vi "Data Log Refresh.vi"(8 "error in (no error)":errorcluster, 11 "Data Cluster":T1) -> (0 "error out":errorcluster)   [LabVIEW 2025]
uses:
  controls/LAB-IQ UI Data.ctl
  Traction Loop/Traction Receipe Enum.ctl
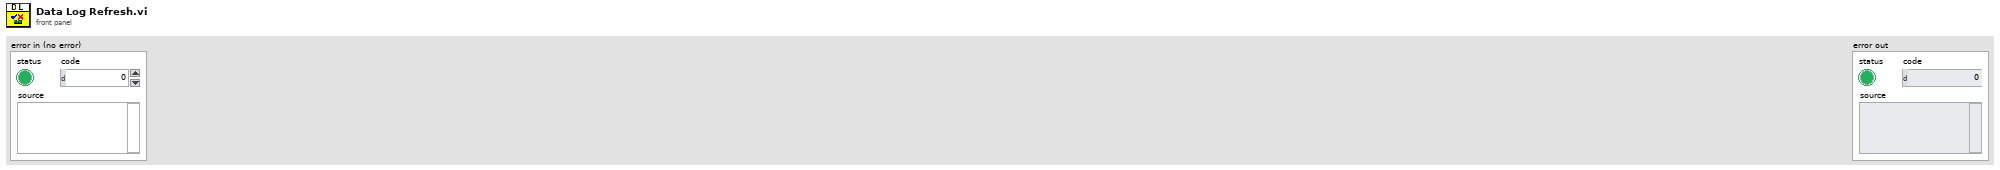
[diagram p1: front panel]
types:
  T1 = typedef "LAB-IQ UI Data.ctl" = cluster{"Main Home Screen":cluster{"GUI":refnum<vi>, "Platform Settings":refnum<vi>, "Configure":refnum<vi>, "Home":refnum<vi>, "EXIT":refnum<vi>, "service 2":refnum<vi>, "MainPage":refnum<vi>, "Analysis":refnum<vi>}, "Platform Settings":cluster{"mm/s  Surge":refnum<vi>, "Drive Error":refnum<vi>, "Disable Axis Jog Soft Limits":refnum<vi>, "mm/s  Sway":refnum<vi>, "Sway and Surge COM Status":refnum<vi>, "Heave COM Status":refnum<vi>, "Enable Platform":refnum<vi>, "Surge Forward Main":refnum<vi>, "Sway Right Main":refnum<vi>, "Sway Left Main":refnum<vi>, "Heave Down Main":refnum<vi>, "Heave Up main":refnum<vi>, "mm/s Heave":refnum<vi>, "mm/sec":refnum<vi>, "mm":refnum<vi>, "Surge Backward Main":refnum<vi>}, "Analysis Screen":cluster{"Analysis Home":refnum<vi>, "Surface Analysis":refnum<vi>, "Imaging":refnum<vi>, "Image Analysis":refnum<vi>, "Post Analysis":refnum<vi>}, "Config Screen":cluster{"Select Load Head":refnum<vi>, "Notes :":refnum<vi>, "FILE":refnum<vi>, "Sample ID :":refnum<vi>, "Operator ID :":refnum<vi>, "Operator Name :":refnum<vi>, "Auto":refnum<vi>}, "Motion Module":cluster{"zNL":refnum<vi>, "NL disp":refnum<vi>, "Rotary Tab":refnum<vi>, "Motion Direction:  3":refnum<vi>, "E.Velocity 2":refnum<vi>, "e.v/ssr 2":refnum<vi>, "Enter Fixed E.Velocity 2":refnum<vi>, "Enter Final SRR 2":refnum<vi>, "Enter initial SRR 2":refnum<vi>, "Enter Fixed SRR 2":refnum<vi>, "Enter the Final E.Velocity (m/s) 2":refnum<vi>, "Enter initial E.Velocity (m/s) 2":refnum<vi>, "Final Speed (RPM) 3":refnum<vi>, "Initial Speed (RPM) 2":refnum<vi>, "Enter the Final Velocity (m/s) 3":refnum<vi>, "Enter initial Velocity (m/s)  3":refnum<vi>, "Ramp Up 2":refnum<vi>, "TEST SELECTION":refnum<vi>, "SPEED SELECTION : ":refnum<vi>, "Angular Oscillation Set":refnum<vi>, "Traction":refnum<vi>, "Step Speed":refnum<vi>, "StepTable For Load-Speed":refnum<vi>, "StepTable For Speed":refnum<vi>, "Surge Forward MM":refnum<vi>, "Surge Backward MM":refnum<vi>, "M3 Image":refnum<vi>, "String 39":refnum<vi>, "Sway Left MM":refnum<vi>, "Sway Right MM":refnum<vi>, "Disable Axis Jog Soft Limits":refnum<vi>, "mm":refnum<vi>, "Heave Down MM":refnum<vi>, "Heave Up MM":refnum<vi>, "Wear Track Diameter (mm)":refnum<vi>, "Set WTD":refnum<vi>, "HomeScratch":refnum<vi>, "HomeRot":refnum<vi>, "PlaceModule":refnum<vi>, "Enter the Angle (Deg)":refnum<vi>, "Enter the Frequency (Hz)":refnum<vi>, "Motion Mode:":refnum<vi>, "LR Sway":refnum<vi>, "Rot Hor":refnum<vi>, "Scratch":refnum<vi>, "LR Cam":refnum<vi>, "MMBack":refnum<vi>, "MMNext":refnum<vi>, "Rot Ver":refnum<vi>, "Rotary Module Selection":refnum<vi>, "calculate rotary":refnum<vi>, "SPEED SELECTION : rotary":refnum<vi>, "Import 2":refnum<vi>, "Save 2":refnum<vi>, "File Path :  2":refnum<vi>, "String 45":refnum<vi>, "StepTable For Speed 3":refnum<vi>, "Enter the Speed(mm/sec)":refnum<vi>, "Enter the Speed(RPM)":refnum<vi>, "Enter Scratch Speed (mm/s):":refnum<vi>, "SwaySpeed Set":refnum<vi>, "Scartch Offset":refnum<vi>, "Motion type:":refnum<vi>, "HomeScratch 2":refnum<vi>, "Enter Scratch length (mm):":refnum<vi>, "Wear Track Diameter":refnum<vi>, "Rotary Speed Exced":refnum<vi>, "Scratch Mode":refnum<vi>, "No of Scratch":refnum<vi>}, "Environmental control":cluster{"Humidity  Status  3":refnum<vi>, "Low Temp  Status  2":refnum<vi>, "TK4 status 2":refnum<vi>, "Stage Temperature":refnum<vi>, "Sample Temperature":refnum<vi>, "Humidity (Amb)":refnum<vi>, "Clear List":refnum<vi>, "Add to list":refnum<vi>, "Wear":refnum<vi>, "Vibration":refnum<vi>, "Humidity (Chamber)":refnum<vi>, "Temperature (Chamber)":refnum<vi>, "ECR ":refnum<vi>, "Temperature (Amb)":refnum<vi>, "Microphone":refnum<vi>, "Acoustic Emission 3":refnum<vi>, "SNext":refnum<vi>, "APBack":refnum<vi>, "Enter the Temperature (°C):":refnum<vi>, "Enter the Stage \nTemperature (°C):":refnum<vi>, "Enter the Humidity (%Rh):":refnum<vi>, "Low Temp":refnum<vi>, "High Temp":refnum<vi>, "Humidity":refnum<vi>, "Sensors Picked":refnum<vi>}, "About Screen":cluster{"Password":refnum<vi>, "Home Service":refnum<vi>, "Advanced Setting":refnum<vi>, "About Tab":refnum<vi>, "ECR Port:":refnum<vi>, "Ramp Port:":refnum<vi>, "Installation/Replacement completed":refnum<vi>, "Loahead":refnum<vi>, "Heave and Surge COM Port:":refnum<vi>, "Sway COM Port:":refnum<vi>, "Temp Modbus:":refnum<vi>, "Humidity Port:":refnum<vi>, "Edit Gain Constants":refnum<vi>, "Save Gain Constants":refnum<vi>}, "Main Screen":cluster{"Main Screen Tab":refnum<vi>, "Angle and Frequency":refnum<vi>, "Stroke (mm)":refnum<vi>, "Angle (Deg)":refnum<vi>, "Main Speed Tab":refnum<vi>, "MTM MOTOR DISPLAY":refnum<vi>, "Disc Speed (m/sec)":refnum<vi>, "Ball Speed (m/sec)":refnum<vi>, "Disc Speed (RPM)":refnum<vi>, "Ball Speed (RPM)":refnum<vi>, "SPEED TAB":refnum<vi>, "Speed (m/sec)":refnum<vi>, "Set Speed (m/sec)":refnum<vi>, "Speed (RPM)":refnum<vi>, "Set Speed":refnum<vi>, "Time Tab":refnum<vi>, "Time ( HH:MM:SS ) 2":refnum<vi>, "Test Duration":refnum<vi>, "Test Duration 4":refnum<vi>, "TEST CYCLE":refnum<vi>, "TOTAL CYCLES":refnum<vi>, "Set Load (N)":refnum<vi>, "Temp Tabs":refnum<vi>, "Heater":refnum<vi>, "TK4 status":refnum<vi>, "ChamberTemp":refnum<vi>, "SetTmp":refnum<vi>, "Controller  Status":refnum<vi>, "ChamberTemp 2":refnum<vi>, "SetTmp 2":refnum<vi>, "Controller  Status 2":refnum<vi>, "ChamberTemp 3":refnum<vi>, "SetTmp 3":refnum<vi>, "Cooling":refnum<vi>, "Load Communication":refnum<vi>, "Ambient \nTemperature":refnum<vi>, "HumCOMStatus":refnum<vi>, "Ambient\n Humidity":refnum<vi>, "Freq (Hz)":refnum<vi>, "Load En":refnum<vi>, "NLt":refnum<vi>, "zNL 2":refnum<vi>, "Humidity On":refnum<vi>, "humidity disp":refnum<vi>, "Set Humidity":refnum<vi>, "NL disp 2":refnum<vi>, "Humidity On 2":refnum<vi>, "humidity disp 2":refnum<vi>, "Set Humidity 2":refnum<vi>, "NL disp 3":refnum<vi>, "AppLoadSeq scratch":refnum<vi>, "Stop Scratch":refnum<vi>, "ClrLog":refnum<vi>, "Trip Log":refnum<vi>, "STOP":refnum<vi>, "Start Test":refnum<vi>, "Test status":refnum<vi>, "AR Led":refnum<vi>, "Data":refnum<vi>, "Health":refnum<vi>, "Sway COM Status":refnum<vi>, "Heave COM Status":refnum<vi>, "Grp Tab":refnum<vi>, "Sub Graph":refnum<vi>, "SD (mm)":refnum<vi>, "Siliding distance Reset Graph":refnum<vi>, "SDGp":refnum<vi>, "Humidity Reset Graph":refnum<vi>, "HumrGp":refnum<vi>, "Acoustic Emission (mV)":refnum<vi>, "Aqucostic Reset Graph":refnum<vi>, "gACQUOS":refnum<vi>, "ECR RESET":refnum<vi>, "ECR":refnum<vi>, "Temperature Reset":refnum<vi>, "Acoustic Emission (mV) 2":refnum<vi>, "Aqucostic Reset Graph 2":refnum<vi>, "gACQUOS 2":refnum<vi>, "ECR RESET 2":refnum<vi>, "ECR 2":refnum<vi>, "Temperature Reset 2":refnum<vi>, "Temperature (deg c)":refnum<vi>, "Speed Reset Graph":refnum<vi>, "Speed Tab":refnum<vi>, "MTM DISC  SPEED":refnum<vi>, "MTM BALL SPEED":refnum<vi>, "speed mm/sec":refnum<vi>, "Hymidity":refnum<vi>, "Humidity Disable trip":refnum<vi>, "CoF Trip  2":refnum<vi>, "Depth Trip":refnum<vi>, "Weart Deapth":refnum<vi>, "Depth Reset Graph":refnum<vi>, "Weart":refnum<vi>, "Depthz":refnum<vi>, "Depth (µm)":refnum<vi>, "WearGp":refnum<vi>, "NL Trip 2":refnum<vi>, "Load pid":refnum<vi>, "Load Disable Trip":refnum<vi>, "Load Reset Graph":refnum<vi>, "NL Display 4":refnum<vi>, "Main Chart 3":refnum<vi>, "BACK":refnum<vi>, "Depth Trip 2":refnum<vi>, "COF TRIP ":refnum<vi>, "Friction Force (N)":refnum<vi>, "FF Reset Graph":refnum<vi>, "FF Disable Trip":refnum<vi>, "FF TRIP":refnum<vi>, "COF Disable Trip":refnum<vi>, "COF Reset Graph":refnum<vi>, "Start Test Temp":refnum<vi>, "zFF":refnum<vi>, "Friction Force (N) Graph":refnum<vi>, "Coefficient of Friction":refnum<vi>, "Scratch Start Test":refnum<vi>, "FF Tab":refnum<vi>, "Cyclic Friction Force (N)":refnum<vi>, "CZ FF":refnum<vi>, "Cyclic Friction Force (N) Graph":refnum<vi>, "Cyclic Coefficient of Friction":refnum<vi>, "Cyclic FF TRIP":refnum<vi>, "Cyclic FF Disable Trip":refnum<vi>, "cyclic COF Disable Trip":refnum<vi>, "cyclic COF TRIP":refnum<vi>, "cyclic COF Reset Graph":refnum<vi>, "Cyclic FF Reset Graph":refnum<vi>, "Test Trip":refnum<vi>, "Multi Scratch Pass":refnum<vi>, "Scratch Start Recording":refnum<vi>}, "Loading":cluster{"Indentation":refnum<vi>, "Reference Sample":refnum<vi>, "Load Cell Communication Slide":refnum<vi>, "com 3":refnum<vi>, "com":refnum<vi>, "DecaForce COM Status":refnum<vi>, "Update":refnum<vi>, "Clear 3":refnum<vi>, "seq":refnum<vi>, "Stribeck table":refnum<vi>, "Stribeck Table  For loading":refnum<vi>, "Loading Mode":refnum<vi>, "Enter the Final Load (N)":refnum<vi>, "Enter the CoF Trip":refnum<vi>, "Enter the Friction Force Trip":refnum<vi>, "Enter the Normal load Trip":refnum<vi>, "Enter the Load  (N)":refnum<vi>, "KiloForce":refnum<vi>, "DecaForce ":refnum<vi>, "MicroForce":refnum<vi>, "LHBack":refnum<vi>, "LHNext":refnum<vi>, "Enter the Loading Rate (N/min)":refnum<vi>, "Message":refnum<vi>, "Warning 2":refnum<vi>, "SSP 0.75":refnum<vi>, "SSP 0.5":refnum<vi>, "SSP 0.3":refnum<vi>, "Warning":refnum<vi>, "gui GIF":refnum<vi>, "Communication is established":refnum<vi>, "AppLoad 4":refnum<vi>, "Multipoint":refnum<vi>, "Load Selection":refnum<vi>}, "PID":cluster{"Ramp":refnum<vi>, "Vertical load (N)":refnum<vi>, "apply load":refnum<vi>, "apply load 2":refnum<vi>, "Enter ByPass Load":refnum<vi>, "Bypass Load":refnum<vi>, "gFF Rot":refnum<vi>}, "Config Parameters":cluster{"Tab Control 3":refnum<vi>, "Tab Control 19":refnum<vi>, "SAMPLES":refnum<vi>, "Re-initilaize":refnum<vi>, "Filter ON/OFF":refnum<vi>, "TracHomeSurgeOffsetCounts 10MM":refnum<vi>, "TracHomeSwayOffsetCounts 10MM":refnum<vi>, "Acoustic Emission:":refnum<vi>, "Apply Filter (FF)":refnum<vi>, "Filter% 2":refnum<vi>, "Apply Filter (Load)":refnum<vi>, "Filter% ":refnum<vi>, "Sway distance (mm)":refnum<vi>, "Surge distance (mm)":refnum<vi>, "DataSavingLoopDelay(ms)":refnum<vi>, "SAVE 2":refnum<vi>, "Enter Distance":refnum<vi>, "Sway Counts:":refnum<vi>, "Distance (mm): 3":refnum<vi>, "Surge Counts:":refnum<vi>, "Distance (mm): 2":refnum<vi>, "Distance (mm):":refnum<vi>, "Heave Counts:":refnum<vi>, "LRMHomeSurgeOffsetCounts":refnum<vi>, "LRMHomeSwayOffsetCounts":refnum<vi>, "TracHomeSurgeOffsetCounts 20MM":refnum<vi>, "TracHomeSwayOffsetCounts 20MM":refnum<vi>, "RotHomeSwayOffsetCounts":refnum<vi>, "RotHomeSurgeOffsetCounts":refnum<vi>, "Heave distance":refnum<vi>, "Zmm":refnum<vi>, "Heave Pulses/mm":refnum<vi>, "Surge Pulses/mm":refnum<vi>, "Sway Pulses/mm":refnum<vi>, "Heave Pitch":refnum<vi>, "Surge Pitch":refnum<vi>, "Sway Pitch":refnum<vi>, "Heave PPR":refnum<vi>, "Surge PPR":refnum<vi>, "Sway PPR":refnum<vi>, "Tab Control 5":refnum<vi>, "Tab Control 14":refnum<vi>, "Tab Control 26":refnum<vi>, "AE":refnum<vi>, "Heave Loop Delay":refnum<vi>, "Heave PID Speed":refnum<vi>, "Surge Jog Speed":refnum<vi>, "Heave Jog Speed":refnum<vi>, "Sway Loop Delay":refnum<vi>, "Sway PID Speed":refnum<vi>, "Sway Jog Speed":refnum<vi>, "DEPTH TRIP VALUE":refnum<vi>, "LOAD TRIP VALUE":refnum<vi>, "DEPTH TRIP   ENABLE":refnum<vi>, "LOAD TRIP  ENABLE":refnum<vi>, "CYCLIC FF TRIP VALUE":refnum<vi>, "FF TRIP VALUE":refnum<vi>, "CYCLIC CoF TRIP VALUE":refnum<vi>, "COF TRIP VALUE":refnum<vi>, "CYCLIC COF TRIP  ENABLE":refnum<vi>, "CYCLIC FF TRIP  ENABLE":refnum<vi>, "FF TRIP  ENABLE":refnum<vi>, "COF TRIP  ENABLE":refnum<vi>, "JOG TRIP LOAD VALUE (N)":refnum<vi>, "Rotary Vertical":refnum<vi>, "Traction":refnum<vi>, "Scratch":refnum<vi>, "LRM CAM":refnum<vi>, "Sway LRM":refnum<vi>, "Rotary Horizontal":refnum<vi>}, "Loading Com Port":cluster{"ClearAll":refnum<vi>, "Mz(Nm)":refnum<vi>, "My(Nm)":refnum<vi>, "Mx(Nm)":refnum<vi>, "Save Dwell":refnum<vi>, "Acq Delay (ms)":refnum<vi>, "Burst Delay (ms)":refnum<vi>, "model":refnum<vi>, "SN":refnum<vi>, "FFx(N)":refnum<vi>, "Sensor IP":refnum<vi>, "Port":refnum<vi>, "FFy(N)":refnum<vi>, "Load(N)":refnum<vi>, "delete Handle":refnum<vi>, "Create Handle":refnum<vi>, "ft_data":refnum<vi>, "ft_range":refnum<vi>, "ft_data 2":refnum<vi>, "stop 6":refnum<vi>, "running_flag":refnum<vi>, "ft_udp_handle":refnum<vi>, "get-data-return":refnum<vi>, "get-range-return":refnum<vi>, "zero-return":refnum<vi>, "filter-return":refnum<vi>, "initial-return":refnum<vi>, "deleteHandle-result":refnum<vi>, "Load Cell Temp":refnum<vi>, "Load Cell":refnum<vi>, "ZeroAll":refnum<vi>, "FORCE (N)":refnum<vi>, "TORQUE (N-m)":refnum<vi>, "Load Cell Link":refnum<vi>}, "Heave AND Surge":cluster{"SURGE POSE":refnum<vi>, "error out Read":refnum<vi>, "HEAVE POSE":refnum<vi>, "State":refnum<vi>, "Homed":refnum<vi>, "Sequence ID":refnum<vi>, "error out Write":refnum<vi>, "faultCode":refnum<vi>, "Ack ID":refnum<vi>, "SPEED":refnum<vi>, "Distance":refnum<vi>, "Mode Command":refnum<vi>, "Heave and Surge Read":refnum<vi>, "Read Heave Temp":refnum<vi>, "Spare 15":refnum<vi>, "Spare 14":refnum<vi>, "Spare 13":refnum<vi>, "Spare 12":refnum<vi>, "Spare 11":refnum<vi>, "Spare 10":refnum<vi>, "Spare 9":refnum<vi>, "Spare 8":refnum<vi>, "Spare 7":refnum<vi>, "Spare 4":refnum<vi>, "Spare 3":refnum<vi>, "Spare 2":refnum<vi>, "Humidity":refnum<vi>, "Temp":refnum<vi>, "Node Id":refnum<vi>, "Spare 1":refnum<vi>, "SPARE 4":refnum<vi>, "SPARE 3":refnum<vi>, "SPARE 2":refnum<vi>, "SPARE 1":refnum<vi>, "fwMajor":refnum<vi>, "fwMinor":refnum<vi>, "Manual Write":refnum<vi>, "Heave and Surge Write":refnum<vi>, "SPARE 5":refnum<vi>, "Reserved ":refnum<vi>, "SPARE 8":refnum<vi>, "SPARE 6":refnum<vi>, "SPARE 7":refnum<vi>, "SPARE 17":refnum<vi>, "SPARE 16":refnum<vi>, "SPARE 15":refnum<vi>, "SPARE 14":refnum<vi>, "SPARE 13":refnum<vi>, "SPARE 12":refnum<vi>, "SPARE 11":refnum<vi>, "SPARE 10":refnum<vi>, "SPARE 9":refnum<vi>, "System UPTIME":refnum<vi>, "Missed Packets":refnum<vi>, "faultCode Surge Right":refnum<vi>, "faultCode Surge Left":refnum<vi>, "faultCode Heave":refnum<vi>, "UPLINK HEAVE":refnum<vi>, "DOWNLINK HEAVE":refnum<vi>}, "New PID LOGIC":cluster{"Fine Tune Zone":refnum<vi>, "PID SDelay":refnum<vi>, "Max_pos_limit":refnum<vi>, "Min_pos_limit":refnum<vi>, "i_limit":refnum<vi>, "pct_scale":refnum<vi>, "Deadband":refnum<vi>, "Kd":refnum<vi>, "Ki":refnum<vi>, "Kp":refnum<vi>, "Current Position":refnum<vi>, "Set Load":refnum<vi>, "Current Load":refnum<vi>, "Pulse delta":refnum<vi>, "Init Step":refnum<vi>, "Max Step Linit":refnum<vi>, "min_deadband_floor":refnum<vi>, "dynamic_spindle_noise_scalar":refnum<vi>, "min_finetune_floor":refnum<vi>, "filter_alpha":refnum<vi>, "PID":refnum<vi>}, "SWAY ":cluster{"fwMajor":refnum<vi>, "Homed":refnum<vi>, "Rotary POSE":refnum<vi>, "State":refnum<vi>, "SWAY POSE":refnum<vi>, "Ack ID":refnum<vi>, "faultCode":refnum<vi>, "Node Id":refnum<vi>, "fwMinor":refnum<vi>, "Spare 6":refnum<vi>, "Spare 5":refnum<vi>, "Spare 4":refnum<vi>, "Spare 3":refnum<vi>, "Spare 2":refnum<vi>, "Spare 1":refnum<vi>, "Spare 7":refnum<vi>, "SPARE  5":refnum<vi>, "error out Write  SWAY ":refnum<vi>, "error out Read SWAY ":refnum<vi>, "Manual Write SWAY ":refnum<vi>, "SWAY WRITE":refnum<vi>, "SPARE  4":refnum<vi>, "SPARE  3":refnum<vi>, "SPARE 2":refnum<vi>, "SPARE 1":refnum<vi>, "Spare 15":refnum<vi>, "Spare 14":refnum<vi>, "Spare 13":refnum<vi>, "Spare 12":refnum<vi>, "Spare 11":refnum<vi>, "Spare 9":refnum<vi>, "Spare 8":refnum<vi>, "SPEED":refnum<vi>, "Distance":refnum<vi>, "Mode Command":refnum<vi>, "Sequence ID":refnum<vi>, "SWAY READ":refnum<vi>, "Spare 10":refnum<vi>, "Read SWAY Temp":refnum<vi>, "faultCode Sway ":refnum<vi>, "Missed Packets":refnum<vi>, "System UPTIME sway":refnum<vi>, "SPARE 6":refnum<vi>, "SPARE 7":refnum<vi>, "SPARE 9":refnum<vi>, "SPARE 11":refnum<vi>, "SPARE 10":refnum<vi>, "SPARE 8":refnum<vi>, "SPARE 13":refnum<vi>, "SPARE 12":refnum<vi>, "SPARE 17":refnum<vi>, "SPARE 16":refnum<vi>, "SPARE 15":refnum<vi>, "SPARE 14":refnum<vi>, "Reserved":refnum<vi>, "faultCode Rotary":refnum<vi>, "UPLINK SWAY":refnum<vi>, "DOWNLINK SWAY":refnum<vi>}, "Analysis Screen":cluster{"Analysis Home":refnum<vi>, "Refresh 2":refnum<vi>, "MEAN 4":refnum<vi>, "SD 4":refnum<vi>, "VARIANCE 4":refnum<vi>, "MEAN  3":refnum<vi>, "SD  3":refnum<vi>, "VARIANCE  3":refnum<vi>, "MEAN 2":refnum<vi>, "SD  2":refnum<vi>, "VARIANCE 2":refnum<vi>, "MEAN":refnum<vi>, "SD":refnum<vi>, "VARIANCE":refnum<vi>, "File 4 Discription":refnum<vi>, "OPEN 4":refnum<vi>, "File Name 4":refnum<vi>, "OPEN 3":refnum<vi>, "File 3 Discription":refnum<vi>, "File Name 3":refnum<vi>, "Y-AXIS":refnum<vi>, "X-AXIS":refnum<vi>, "XY Graph":refnum<vi>, "File Name 2":refnum<vi>, "File Name 1":refnum<vi>, "OPEN 2":refnum<vi>, "OPEN 1":refnum<vi>, "File 1 Discription ":refnum<vi>, "File 2 Discription":refnum<vi>, "Export":refnum<vi>, "File Format":refnum<vi>}, "Traction":cluster{"faultCode Traction 2":refnum<vi>, "faultCode Traction 1":refnum<vi>, "Missed Packets":refnum<vi>, "System UPTIME Traction":refnum<vi>, "SPARE 17":refnum<vi>, "SPARE 16":refnum<vi>, "SPARE 15":refnum<vi>, "SPARE 14":refnum<vi>, "SPARE 13":refnum<vi>, "SPARE 12":refnum<vi>, "SPARE 11":refnum<vi>, "SPARE 10":refnum<vi>, "SPARE 9":refnum<vi>, "SPARE 8":refnum<vi>, "SPARE 7":refnum<vi>, "SPARE 6":refnum<vi>, "Reserved":refnum<vi>, "SPARE  5":refnum<vi>, "Manual Write TRACTION":refnum<vi>, "TRACTION WRITE":refnum<vi>, "SPARE  4":refnum<vi>, "SPARE  3":refnum<vi>, "SPARE 2":refnum<vi>, "SPARE 1":refnum<vi>, "Spare 7":refnum<vi>, "Spare 6":refnum<vi>, "Spare 5":refnum<vi>, "Spare 4":refnum<vi>, "Spare 2":refnum<vi>, "Spare 1":refnum<vi>, "Node Id":refnum<vi>, "Read TRACTION Temp":refnum<vi>, "fwMinor":refnum<vi>, "fwMajor":refnum<vi>, "faultCode":refnum<vi>, "TRACTION POSE":refnum<vi>, "TRACTION POSE 2":refnum<vi>, "Homed":refnum<vi>, "State":refnum<vi>, "Ack ID":refnum<vi>, "SPEED":refnum<vi>, "Distance":refnum<vi>, "Mode Command":refnum<vi>, "Sequence ID":refnum<vi>, "error out Read TRACTION":refnum<vi>, "error out Write  TRACTION":refnum<vi>, "TRACTION READ":refnum<vi>, "Spare 3":refnum<vi>, "Downlink traction":refnum<vi>, "Uplink Traction":refnum<vi>}, "Traction reciepe":cluster{"SRR Sweep Range (%) Stribeck":refnum<vi>, "Traction Receipe":refnum<vi>, "Total Execution Time":refnum<vi>, "Total Steps":refnum<vi>, "Duration / Step (s)  Stribeck":refnum<vi>, "STRIBECK Fixed SRR List (%)":refnum<vi>, "Duration / Step (s) Traction":refnum<vi>, "SRR Sweep Range (%) traction":refnum<vi>, "Rolling Speed (mm/s)":refnum<vi>, "Temperature Stages (°C)":refnum<vi>, "Ball Load (N)":refnum<vi>, "Lubricant Name":refnum<vi>, "Profile File Name":refnum<vi>, "SET entrainment Velocity":refnum<vi>, "Test Array Size":refnum<vi>, "SRR INDEX [ STRIBECK]":refnum<vi>, "Stribeck Size":refnum<vi>, "SET SRR":refnum<vi>, "ELAPSED TIMER ":refnum<vi>, "BALL SET RPM":refnum<vi>, "DISC SET RPM":refnum<vi>, "SET LOAD":refnum<vi>, "TEMPERATURE READ":refnum<vi>, "SET TEMPERATURE":refnum<vi>, "Traction Size":refnum<vi>, "DISC SPEED (rpm)":refnum<vi>, "BALL SPEED (rpm)":refnum<vi>, "BALL WEAR TRACK":refnum<vi>, "DISC WEARTRACK":refnum<vi>, "SRR INDEX [ TRACTION]":refnum<vi>, "Start Index Type":refnum<vi>, "Enum - Menu":refnum<vi>, "Ball (mm/sec)":refnum<vi>, "Disc (mm/sec)":refnum<vi>}, "Traction Control":cluster{"HomeTraction":refnum<vi>, "Demo Mode Display":refnum<vi>, "Traction Message":refnum<vi>, "Traction Step Update Details":refnum<vi>, "Main Tab sequence for selection":refnum<vi>, "Ramp Tab":refnum<vi>, "e.v/ssr":refnum<vi>, "Enter Fixed E.Velocity":refnum<vi>, "Enter Final SRR":refnum<vi>, "Enter initial SRR":refnum<vi>, "Enter Fixed SRR":refnum<vi>, "Enter the Final E.Velocity (m/s)":refnum<vi>, "Enter initial E.Velocity (m/s)":refnum<vi>, "Ball WTD":refnum<vi>, "E.Velocity":refnum<vi>, "Enter the Final Velocity (m/s)":refnum<vi>, "Enter initial Velocity (m/s)":refnum<vi>, "Ramp Up   Disc":refnum<vi>, "Initial DiscSpeed (RPM)":refnum<vi>, "Final Speed (RPM) Ball":refnum<vi>, "Final Speed (RPM)":refnum<vi>, "Initial Speed (RPM) Ball":refnum<vi>, "Enter the Final Velocity (m/s) Ball":refnum<vi>, "Enter initial Velocity (m/s) Ball":refnum<vi>, "Ramp Up":refnum<vi>, "ExceedBallSpeed step":refnum<vi>, "ExceedDiscSpeed":refnum<vi>, "BallSpeed Exceed Indication":refnum<vi>, "Apply":refnum<vi>, "SPEED SELECTION : MTM":refnum<vi>, "SPEED SELECTION : MTM 2":refnum<vi>, "TEST SELECTION (MTM)":refnum<vi>, "MTM Test Selection":refnum<vi>, "File Path Tab":refnum<vi>, "File Path String":refnum<vi>, "Save":refnum<vi>, "Save  2":refnum<vi>, "Import ":refnum<vi>, "File Path :":refnum<vi>, "Step Sequence Indication Tab":refnum<vi>, "Step Sequence Indication":refnum<vi>, "Calculate Step":refnum<vi>, "StepTable":refnum<vi>, "ExceedDiscSpeed  Cinstant Speed":refnum<vi>, "ExceedBallSpeed Constant":refnum<vi>, "TEST SELECTION (MTM) 2":refnum<vi>, "SPEED SELECTION : MTM 3":refnum<vi>, "MTM Test Selection 2":refnum<vi>, "Enter the Speed (m/sec): ":refnum<vi>, "Enter the Speed (m/sec):  2":refnum<vi>, "Enter the Speed (RPM):":refnum<vi>, "Lower Spped ":refnum<vi>, "Upper":refnum<vi>, "Enter the Speed (RPM):Ball":refnum<vi>, "Disc Motion Direction: ":refnum<vi>, "Ball Motion Direction :":refnum<vi>, "Motion Mode: ":refnum<vi>, "Wear Track Diameter (mm) ":refnum<vi>, "Disc Speed Indicator":refnum<vi>, "ExceedBallSpeed":refnum<vi>}, "Acquostic":cluster{"Last Config Rejected ":refnum<vi>, "rx command count":refnum<vi>, "Current Filter Id":refnum<vi>, "Isolated Gain":refnum<vi>, "DAQ Status":refnum<vi>, "error out":refnum<vi>, "error in (no error)":refnum<vi>, "Uplink Packet":refnum<vi>, "data out":refnum<vi>, "Downlink Packet":refnum<vi>, "Gains":refnum<vi>, "Manual Write Acquostic":refnum<vi>, "Acoustic Graphs":refnum<vi>}}
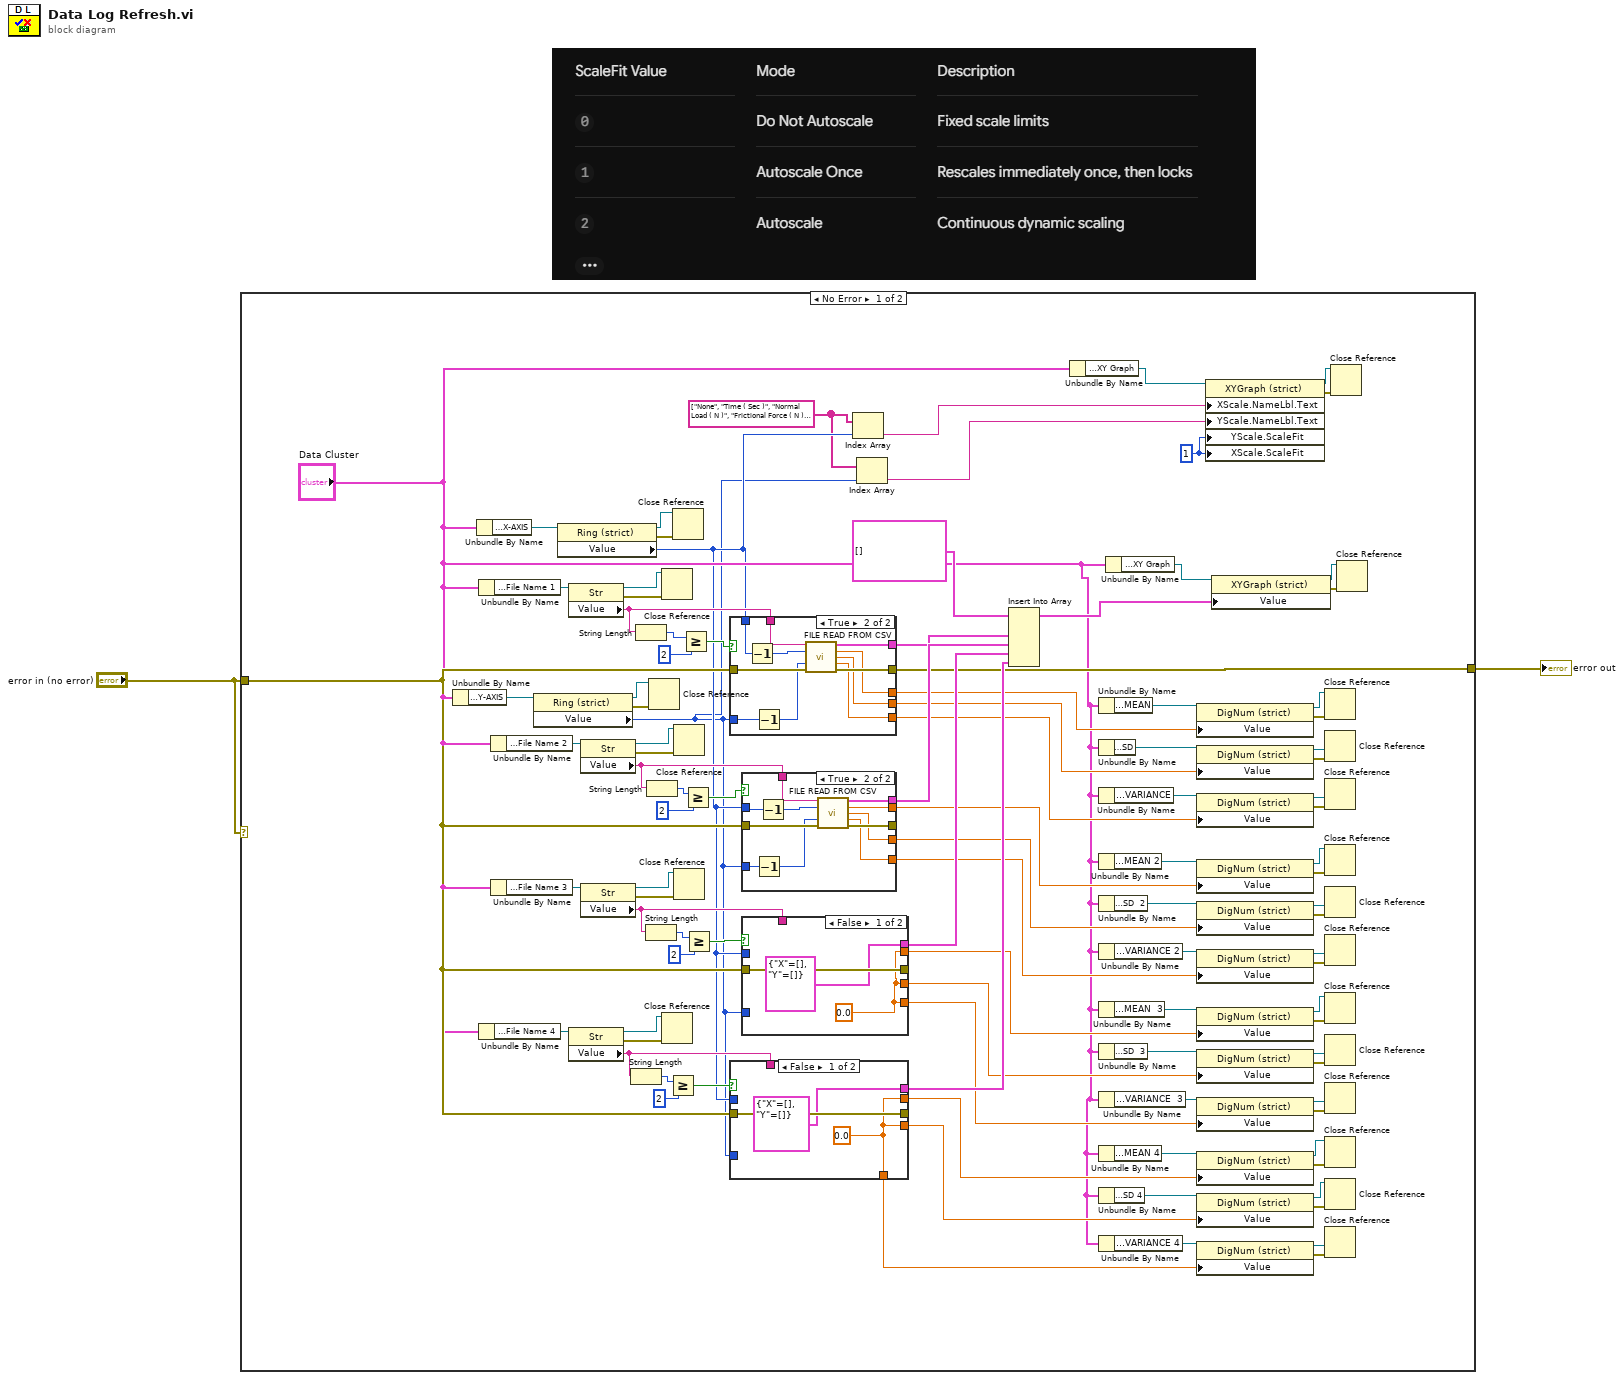
[diagram p0: block diagram]
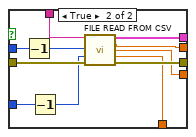
[diagram p2: hidden frame]
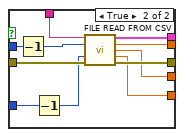
[diagram p3: hidden frame]
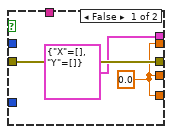
[diagram p4: hidden frame]
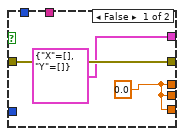
[diagram p5: hidden frame]
diagram:
  n1 = case shown="No Error" "error in (no error)" {
    tunnel: "error in (no error)" -> [w90 _]
    tunnel: [w64 _] -> w2
    frame No Error {
      w3 = u8 1 ("X Scale.Scale Fit")
      w6 = string[] ["None", "Time ( Sec )", "Normal Load ( N )", "Frictional Force ( N )", "Coefficient of Friction", "Depth ( Microns )", "Speed ( RPM )", "Frequency ( Hz )", "Angle ( Degree )", "Cyclic Friction Force ( N )", "Cyclic Co efficient Friction ", "Stage temperature ( Degree celcius )", "Sample temperature ( Degree celcius )", "Stroke Length ( mm )", "Scratch Speed ( mm/sec )", "Amb Humidity ( % Rh ) ", "Amb Temperature (Deg C)", "Acoustic (mV)", "Mx (Nm)", "My (Nm)", "Mz (Nm)", "Humidity ( % Rh )", "Sliding Distance (mm)", "Wear Track Diameter (mm)", "Fx(N)", "Fy(N)", "MTM BallSpeed (RPM)", "MTM DiscSpeed (RPM)", "Entrainment Speed", "Slide Role", "Slip(%)", "Rotary Speed (m/sec)", "MTM Ball Speed (m/sec)", "MTM Disc Speed (m/sec)", "ECR (ohms)"] ("Strings []")
      n2 = Unbundle By Name("Data Cluster") -> ("Analysis Screen.Y-AXIS"=w103:refnum<vi>)
      n3 = Unbundle By Name("Data Cluster") -> ("Analysis Screen.X-AXIS"=w100:refnum<vi>)
      n4 = Unbundle By Name("Data Cluster") -> ("Analysis Screen.File Name 1"=w62:refnum<vi>)
      n5 = Unbundle By Name("Data Cluster") -> ("Analysis Screen.File Name 4"=w84:refnum<vi>)
      n6 = Unbundle By Name("Data Cluster") -> ("Analysis Screen.File Name 2"=w74:refnum<vi>)
      n7 = Unbundle By Name("Data Cluster") -> ("Analysis Screen.File Name 3"=w77:refnum<vi>)
      n8 = property class="Ring (strict)"(reference=w103) -> (reference out=w105:refnum<vi>, error out=w104:errorcluster, "Value"=w5:u16)  [unwired: 1 in]
      n9 = property class="Ring (strict)"(reference=w100) -> (reference out=w102:refnum<vi>, error out=w101:errorcluster, "Value"=w8:u16)  [unwired: 1 in]
      n10 = property class="Str"(reference=w62) -> (reference out=w61:refnum<vi>, error out=w63:errorcluster, "Value"=w65:string)  [unwired: 1 in]
      n11 = property class="Str"(reference=w84) -> (reference out=w83:refnum<vi>, error out=w85:errorcluster, "Value"=w86:string)  [unwired: 1 in]
      n12 = property class="Str"(reference=w74) -> (reference out=w75:refnum<vi>, error out=w73:errorcluster, "Value"=w72:string)  [unwired: 1 in]
      n13 = property class="Str"(reference=w77) -> (reference out=w76:refnum<vi>, error out=w78:errorcluster, "Value"=w79:string)  [unwired: 1 in]
      n14 = String Length(string=w86) -> (length=w87:i32)
      n15 = String Length(string=w65) -> (length=w66:i32)
      n16 = String Length(string=w79) -> (length=w80:i32)
      n17 = String Length(string=w72) -> (length=w71:i32)
      n18 = Close Reference(reference=w105, error in (no error)=w104) -> ()  [unwired: 1 out]
      n19 = Close Reference(reference=w61, error in (no error)=w63) -> ()  [unwired: 1 out]
      n20 = Close Reference(reference=w83, error in (no error)=w85) -> ()  [unwired: 1 out]
      n21 = Greater Or Equal?(x=w87, y=2) -> (x >= y?=w89:bool)
      n22 = Close Reference(reference=w102, error in (no error)=w101) -> ()  [unwired: 1 out]
      n23 = Close Reference(reference=w75, error in (no error)=w73) -> ()  [unwired: 1 out]
      n24 = Close Reference(reference=w76, error in (no error)=w78) -> ()  [unwired: 1 out]
      n25 = Greater Or Equal?(x=w66, y=2) -> (x >= y?=w68:bool)
      n26 = Greater Or Equal?(x=w71, y=2) -> (x >= y?=w69:bool)
      n27 = Greater Or Equal?(x=w80, y=2) -> (x >= y?=w82:bool)
      n28 = case shown="True" w68 {
        tunnel: w90 -> [w150 w161]
        tunnel: [w150 w160] -> w64
        tunnel: w65 -> [_ w159]
        tunnel: [cluster{"X":dbl[], "Y":dbl[]} {"X"=[], "Y"=[]} ("output cluster") w158] -> w95
        tunnel: w8 -> [_ w157]
        tunnel: w5 -> [_ w156]
        tunnel: [w148 w153] -> w51
        tunnel: [w148 w152] -> w50
        tunnel: [w148 w151] -> w49
        frame False {
          w148 = 0.0
        }
        frame True {
          n29 = Decrement(x=w157) -> (x-1=w155:u16)
          n30 = Decrement(x=w156) -> (x-1=w154:u16)
          n31 = call "FILE READ FROM CSV.vi"("File Path"=w159, "X-AXIS"=w155, "Y-AXIS"=w154, "error in (no error)"=w161) -> ("output cluster"=w158:cluster{"X":dbl[], "Y":dbl[]}, "mean"=w153:dbl, "standard deviation"=w152:dbl, "variance"=w151:dbl, "error out"=w160:errorcluster)  [unwired: 7 in]
        }
      }
      n32 = case shown="False" w89 {
        tunnel: w90 -> [w108 w119]
        tunnel: [w108 w118] -> _
        tunnel: w86 -> [_ w117]
        tunnel: [cluster{"X":dbl[], "Y":dbl[]} {"X"=[], "Y"=[]} ("output cluster") w116] -> w98
        tunnel: w8 -> [_ w115]
        tunnel: w5 -> [_ w113]
        tunnel: [w106 w111] -> w15
        tunnel: [w106 w110] -> w14
        tunnel: [w106 w109] -> w13
        frame False {
          w106 = 0.0
        }
        frame True {
          n33 = Decrement(x=w115) -> (x-1=w114:u16)
          n34 = Decrement(x=w113) -> (x-1=w112:u16)
          n35 = call "FILE READ FROM CSV.vi"("File Path"=w117, "X-AXIS"=w114, "Y-AXIS"=w112, "error in (no error)"=w119) -> ("output cluster"=w116:cluster{"X":dbl[], "Y":dbl[]}, "mean"=w111:dbl, "standard deviation"=w110:dbl, "variance"=w109:dbl, "error out"=w118:errorcluster)  [unwired: 7 in]
        }
      }
      n36 = case shown="True" w69 {
        tunnel: w90 -> [w136 w147]
        tunnel: [w136 w146] -> _
        tunnel: w72 -> [_ w145]
        tunnel: [cluster{"X":dbl[], "Y":dbl[]} {"X"=[], "Y"=[]} ("output cluster") w144] -> w96
        tunnel: w8 -> [_ w143]
        tunnel: w5 -> [_ w141]
        tunnel: [w134 w139] -> w39
        tunnel: [w134 w138] -> w38
        tunnel: [w134 w137] -> w37
        frame False {
          w134 = 0.0
        }
        frame True {
          n37 = Decrement(x=w141) -> (x-1=w140:u16)
          n38 = Decrement(x=w143) -> (x-1=w142:u16)
          n39 = call "FILE READ FROM CSV.vi"("File Path"=w145, "X-AXIS"=w142, "Y-AXIS"=w140, "error in (no error)"=w147) -> ("output cluster"=w144:cluster{"X":dbl[], "Y":dbl[]}, "mean"=w139:dbl, "standard deviation"=w138:dbl, "variance"=w137:dbl, "error out"=w146:errorcluster)  [unwired: 7 in]
        }
      }
      n40 = case shown="False" w82 {
        tunnel: w90 -> [w122 w133]
        tunnel: [w122 w132] -> _
        tunnel: w79 -> [_ w131]
        tunnel: [cluster{"X":dbl[], "Y":dbl[]} {"X"=[], "Y"=[]} ("output cluster") w130] -> w97
        tunnel: w8 -> [_ w129]
        tunnel: w5 -> [_ w127]
        tunnel: [w120 w125] -> w27
        tunnel: [w120 w124] -> w26
        tunnel: [w120 w123] -> w25
        frame False {
          w120 = 0.0
        }
        frame True {
          n41 = Decrement(x=w129) -> (x-1=w128:u16)
          n42 = Decrement(x=w127) -> (x-1=w126:u16)
          n43 = call "FILE READ FROM CSV.vi"("File Path"=w131, "X-AXIS"=w128, "Y-AXIS"=w126, "error in (no error)"=w133) -> ("output cluster"=w130:cluster{"X":dbl[], "Y":dbl[]}, "mean"=w125:dbl, "standard deviation"=w124:dbl, "variance"=w123:dbl, "error out"=w132:errorcluster)  [unwired: 7 in]
        }
      }
      n44 = Index Array(array=w6, index=w8) -> (element=w7:string)
      n45 = Index Array(array=w6, index=w5) -> (element=w4:string)
      n46 = Insert Into Array(array=cluster{"Array 2":dbl[], "Array 2":dbl[]}[] [] ("Value"), new element #1=w95, new element #2=w96, new element #3=w97, new element #4=w98) -> (w99:cluster{"Array 2":dbl[], "Array 2":dbl[]}[])  [unwired: 1 in]
      n47 = Unbundle By Name("Data Cluster") -> ("Analysis Screen.XY Graph"=w11:refnum<vi>)
      n48 = Unbundle By Name("Data Cluster") -> ("Analysis Screen.MEAN"=w59:refnum<vi>)
      n49 = Unbundle By Name("Data Cluster") -> ("Analysis Screen.SD"=w56:refnum<vi>)
      n50 = Unbundle By Name("Data Cluster") -> ("Analysis Screen.VARIANCE"=w53:refnum<vi>)
      n51 = Unbundle By Name("Data Cluster") -> ("Analysis Screen.MEAN 2"=w41:refnum<vi>)
      n52 = Unbundle By Name("Data Cluster") -> ("Analysis Screen.SD  2"=w44:refnum<vi>)
      n53 = Unbundle By Name("Data Cluster") -> ("Analysis Screen.VARIANCE 2"=w47:refnum<vi>)
      n54 = Unbundle By Name("Data Cluster") -> ("Analysis Screen.MEAN  3"=w35:refnum<vi>)
      n55 = Unbundle By Name("Data Cluster") -> ("Analysis Screen.SD  3"=w32:refnum<vi>)
      n56 = Unbundle By Name("Data Cluster") -> ("Analysis Screen.VARIANCE  3"=w29:refnum<vi>)
      n57 = Unbundle By Name("Data Cluster") -> ("Analysis Screen.MEAN 4"=w17:refnum<vi>)
      n58 = Unbundle By Name("Data Cluster") -> ("Analysis Screen.SD 4"=w20:refnum<vi>)
      n59 = Unbundle By Name("Data Cluster") -> ("Analysis Screen.VARIANCE 4"=w23:refnum<vi>)
      n60 = Unbundle By Name("Data Cluster") -> ("Analysis Screen.XY Graph"=w92:refnum<vi>)
      n61 = property class="DigNum (strict)"(reference=w59, "Value"=w51) -> (reference out=w58:refnum<vi>, error out=w60:errorcluster)  [unwired: 1 in]
      n62 = property class="DigNum (strict)"(reference=w56, "Value"=w50) -> (reference out=w57:refnum<vi>, error out=w55:errorcluster)  [unwired: 1 in]
      n63 = property class="DigNum (strict)"(reference=w53, "Value"=w49) -> (reference out=w52:refnum<vi>, error out=w54:errorcluster)  [unwired: 1 in]
      n64 = property class="DigNum (strict)"(reference=w41, "Value"=w39) -> (reference out=w42:refnum<vi>, error out=w40:errorcluster)  [unwired: 1 in]
      n65 = property class="DigNum (strict)"(reference=w44, "Value"=w38) -> (reference out=w43:refnum<vi>, error out=w45:errorcluster)  [unwired: 1 in]
      n66 = property class="DigNum (strict)"(reference=w47, "Value"=w37) -> (reference out=w48:refnum<vi>, error out=w46:errorcluster)  [unwired: 1 in]
      n67 = property class="DigNum (strict)"(reference=w35, "Value"=w27) -> (reference out=w34:refnum<vi>, error out=w36:errorcluster)  [unwired: 1 in]
      n68 = property class="DigNum (strict)"(reference=w32, "Value"=w26) -> (reference out=w33:refnum<vi>, error out=w31:errorcluster)  [unwired: 1 in]
      n69 = property class="DigNum (strict)"(reference=w29, "Value"=w25) -> (reference out=w28:refnum<vi>, error out=w30:errorcluster)  [unwired: 1 in]
      n70 = property class="DigNum (strict)"(reference=w17, "Value"=w15) -> (reference out=w18:refnum<vi>, error out=w16:errorcluster)  [unwired: 1 in]
      n71 = property class="DigNum (strict)"(reference=w20, "Value"=w14) -> (reference out=w19:refnum<vi>, error out=w21:errorcluster)  [unwired: 1 in]
      n72 = property class="DigNum (strict)"(reference=w23, "Value"=w13) -> (reference out=w24:refnum<vi>, error out=w22:errorcluster)  [unwired: 1 in]
      n73 = property class="XYGraph (strict)"(reference=w11, "XScale.NameLbl.Text"=w7, "YScale.NameLbl.Text"=w4, "YScale.ScaleFit"=w3, "XScale.ScaleFit"=w3) -> (reference out=w12:refnum<vi>, error out=w10:errorcluster)  [unwired: 1 in]
      n74 = property class="XYGraph (strict)"(reference=w92, "Value"=w99) -> (reference out=w91:refnum<vi>, error out=w93:errorcluster)  [unwired: 1 in]
      n75 = Close Reference(reference=w58, error in (no error)=w60) -> ()  [unwired: 1 out]
      n76 = Close Reference(reference=w57, error in (no error)=w55) -> ()  [unwired: 1 out]
      n77 = Close Reference(reference=w52, error in (no error)=w54) -> ()  [unwired: 1 out]
      n78 = Close Reference(reference=w42, error in (no error)=w40) -> ()  [unwired: 1 out]
      n79 = Close Reference(reference=w43, error in (no error)=w45) -> ()  [unwired: 1 out]
      n80 = Close Reference(reference=w48, error in (no error)=w46) -> ()  [unwired: 1 out]
      n81 = Close Reference(reference=w34, error in (no error)=w36) -> ()  [unwired: 1 out]
      n82 = Close Reference(reference=w33, error in (no error)=w31) -> ()  [unwired: 1 out]
      n83 = Close Reference(reference=w28, error in (no error)=w30) -> ()  [unwired: 1 out]
      n84 = Close Reference(reference=w18, error in (no error)=w16) -> ()  [unwired: 1 out]
      n85 = Close Reference(reference=w19, error in (no error)=w21) -> ()  [unwired: 1 out]
      n86 = Close Reference(reference=w24, error in (no error)=w22) -> ()  [unwired: 1 out]
      n87 = Close Reference(reference=w12, error in (no error)=w10) -> ()  [unwired: 1 out]
      n88 = Close Reference(reference=w91, error in (no error)=w93) -> ()  [unwired: 1 out]
    }
    frame Error {
    }
  }
  "error out" <- w2
